vi "example_detect_boolean_edges_1.vi"() -> ()   [LabVIEW 2015]
uses:
  polys/poly_detect_boolean_edges_falling.vi
  polys/poly_detect_boolean_edges_both.vi
  polys/poly_detect_boolean_edges_rising.vi
  cores/core_detect_boolean_edges.vi
  <vilib>/ptbypt/NI_PtbyPt.lvlib
panel:
  out "any":bool
  out "falling":bool
  out "rising":bool
  out "graph":T1(graph) caption="random boolean sequence"
  in  "stop":bool
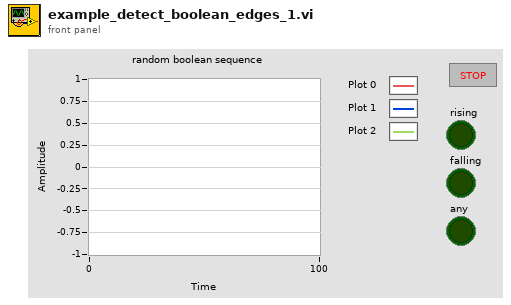
[diagram p1: front panel]
types:
  T1 = cluster{"number: 0 to 1":dbl, "threshold":dbl, i16}
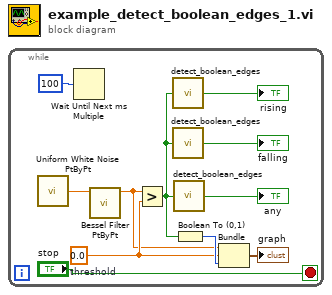
[diagram p0: block diagram]
diagram:
  n1 = while {
    stop <- "stop" stop-if-true
    w7 = 0.0  # threshold
    n2 = call <vilib>:"Uniform White Noise PtByPt.vi"() -> ("uniform white noise"=w1:dbl)  [unwired: 3 in]
    n3 = Wait Until Next ms Multiple(millisecond multiple=u32 100 ("milliseconds to wait")) -> ()  [unwired: 1 out]
    n4 = call <vilib>:"Bessel Filter PtByPt.vi"("x"=w1) -> ("Filtered x"=w2:dbl)  [unwired: 8 in, 1 out]
    n5 = Greater?(x=w2, y=w7) -> (0:w6:bool)
    n6 = call-poly "detect_boolean_edges.vi"("tf input"=w6) -> ("rising edge"=→"rising":bool)  [unwired: 4 in]
    n7 = call-poly "detect_boolean_edges.vi"("tf input"=w6) -> ("falling edge"=→"falling":bool)  [unwired: 4 in]
    n8 = call-poly "detect_boolean_edges.vi"("tf input"=w6) -> ("edge"=→"any":bool)  [unwired: 4 in]
    n9 = Boolean To (0,1)(Boolean=w6) -> (0, 1=w9:i16)
    n10 = Bundle("Filtered x"=w2, "threshold"=w7, w9) -> (→"graph":cluster{"Filtered x":dbl, "threshold":dbl, i16})  [unwired: 1 in]
  }
